vi "CRYCheck Operation.vi"(8 "Operation":string, 10 "Item Symbols In":i32[](array[numeric]), 11 "Index Array In":i32[](array[numeric])) -> (1 "Operation ?":bool, 2 "Item Symbols Out":i32[](array[numeric]), 3 "Array Out":i32[](array[numeric]))   [LabVIEW 2013]
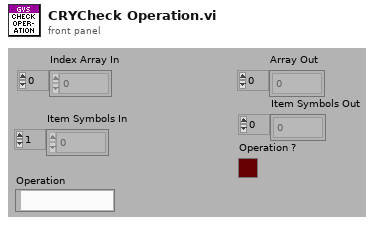
[diagram p1: front panel]
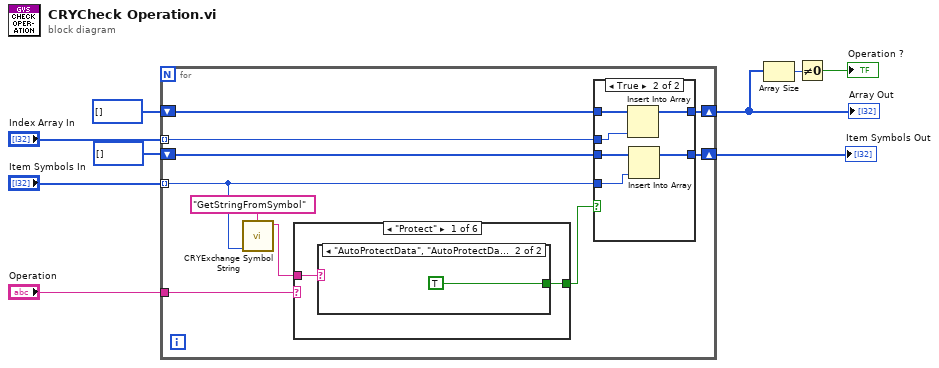
[diagram p0: block diagram]
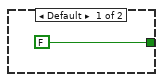
[diagram p2: hidden frame]
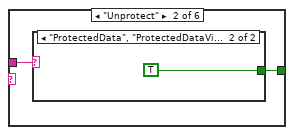
[diagram p3: hidden frame]
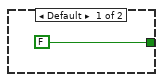
[diagram p4: hidden frame]
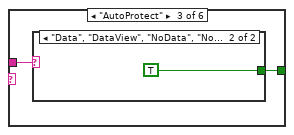
[diagram p5: hidden frame]
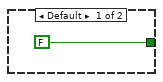
[diagram p6: hidden frame]
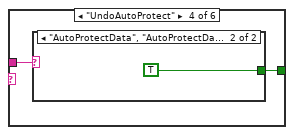
[diagram p7: hidden frame]
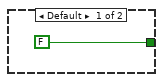
[diagram p8: hidden frame]
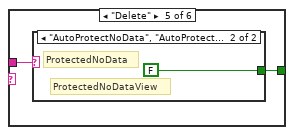
[diagram p9: hidden frame]
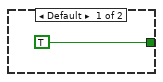
[diagram p10: hidden frame]
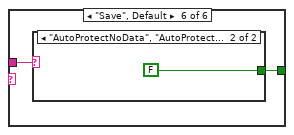
[diagram p11: hidden frame]
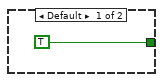
[diagram p12: hidden frame]
diagram:
  n1 = for {
    tunnel: "Index Array In" -> [w17] mode=indexing
    tunnel: "Item Symbols In" -> [w11] mode=indexing
    shift-right: [w18] -> w5
    shift-left: i32[] [] ("Index Array Out") -> [w19]
    tunnel: "Operation" -> [w13]
    shift-right: [w16] -> w1
    shift-left: i32[] [] ("Item Symbols In") -> [w15]
    n2 = call "CRYExchange Symbol String.vi"("nData"=w11, "sAction"="GetStringFromSymbol") -> ("sData out"=w12:string)  [unwired: 8 in, 1 out]
    n3 = case shown="\"Protect\"" w13 {
      tunnel: w12 -> [w21 w25 w29 w33 w37 w41]
      tunnel: [w20 w24 w28 w32 w36 w40] -> w10
      frame "Protect" {
        n4 = case shown="\"AutoProtectData\", \"AutoProtectDataView\", \"Data\", \"DataView\"" w21 {
          tunnel: [FALSE ("x = y?") TRUE ("x = y?")] -> w20
          frame Default {
          }
          frame "AutoProtectData", "AutoProtectDataView", "Data", "DataView" {
          }
        }
      }
      frame "Unprotect" {
        n5 = case shown="\"ProtectedData\", \"ProtectedDataView\", \"ProtectedNoData\", \"ProtectedNoDataView\"" w25 {
          tunnel: [FALSE ("x = y?") TRUE ("x = y?")] -> w24
          frame Default {
          }
          frame "ProtectedData", "ProtectedDataView", "ProtectedNoData", "ProtectedNoDataView" {
          }
        }
      }
      frame "AutoProtect" {
        n6 = case shown="\"Data\", \"DataView\", \"NoData\", \"NoDataView\"" w29 {
          tunnel: [FALSE ("x = y?") TRUE ("x = y?")] -> w28
          frame Default {
          }
          frame "Data", "DataView", "NoData", "NoDataView" {
          }
        }
      }
      frame "UndoAutoProtect" {
        n7 = case shown="\"AutoProtectData\", \"AutoProtectDataView\", \"AutoProtectNoData\", \"AutoProtectNoDataView\"" w33 {
          tunnel: [FALSE ("x = y?") TRUE ("x = y?")] -> w32
          frame Default {
          }
          frame "AutoProtectData", "AutoProtectDataView", "AutoProtectNoData", "AutoProtectNoDataView" {
          }
        }
      }
      frame "Delete" {
        n8 = case shown="\"AutoProtectNoData\", \"AutoProtectNoDataView\", \"NoData\", \"NoDataView\"" w37 {
          tunnel: [TRUE ("x = y?") FALSE ("x = y?")] -> w36
          frame Default {
          }
          frame "AutoProtectNoData", "AutoProtectNoDataView", "NoData", "NoDataView" {
            # "ProtectedNoDataView"
            # "ProtectedNoData"
          }
        }
      }
      frame "Save", Default {
        n9 = case shown="\"AutoProtectNoData\", \"AutoProtectNoDataView\", \"NoData\", \"NoDataView\", \"ProtectedNoData\", \"ProtectedNoDataView\"" w41 {
          tunnel: [TRUE ("x = y?") FALSE ("x = y?")] -> w40
          frame Default {
          }
          frame "AutoProtectNoData", "AutoProtectNoDataView", "NoData", "NoDataView", "ProtectedNoData", "ProtectedNoDataView" {
          }
        }
      }
    }
    n10 = case shown="True" w10 {
      tunnel: w19 -> [w45 w51]
      tunnel: [w45 w50] -> w18
      tunnel: w17 -> [_ w49]
      tunnel: w15 -> [w44 w48]
      tunnel: w11 -> [_ w47]
      tunnel: [w44 w46] -> w16
      frame False {
      }
      frame True {
        n11 = Insert Into Array(array=w51, new element=w49) -> (w50:i32[])  [unwired: 1 in]
        n12 = Insert Into Array(array=w48, new element=w47) -> (w46:i32[])  [unwired: 1 in]
      }
    }
  }
  "Array Out" <- w5
  "Item Symbols Out" <- w1
  n13 = Array Size(array=w5) -> (size(s)=w6:i32)
  n14 = Not Equal To 0?(x=w6) -> (x != 0?=→"Operation ?":bool)
